vi "Set_Response_Type.vi"(8 "error in (no error)":errorcluster, 11 "OAuth in":refnum<class "OAuth.lvclass">) -> (0 "error out":errorcluster, 3 "OAuth out":refnum<class "OAuth.lvclass">)   [LabVIEW 2016, in "OAuth.lvclass"]
uses:
  OAuth.lvclass
  OAuth.lvclass/OAuth.ctl
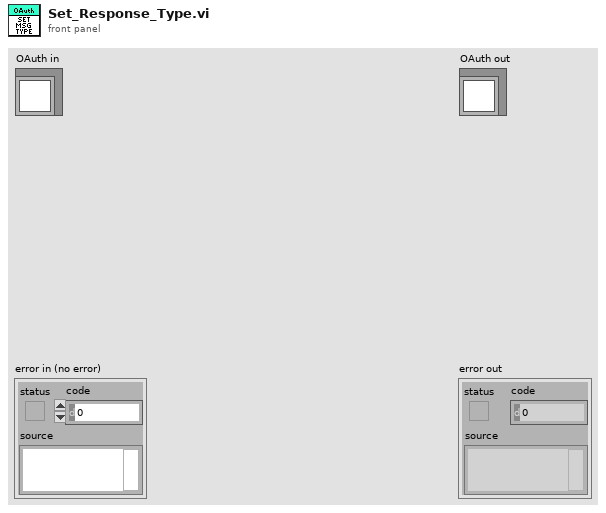
[diagram p1: front panel]
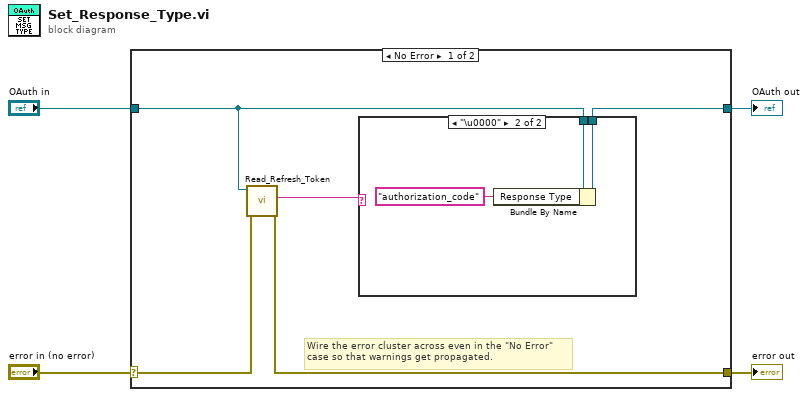
[diagram p0: block diagram]
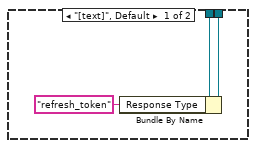
[diagram p2: hidden frame]
diagram:
  n1 = case shown="No Error" "error in (no error)" {
    selector: "error in (no error)" -> [w8 w17]
    tunnel: [w7 w17] -> w3
    tunnel: [w5 w16] -> w1
    tunnel: "OAuth in" -> [w6 w16]
    frame No Error {
      # "Wire the error cluster across even in the \"No Error\"\ncase so that warnings get propagated."
      n2 = call-dynamic "Read_Refresh_Token.vi"("error in (no error)"=w8, "OAuth in"=w6) -> ("error out"=w7:errorcluster, "String"=w9:string)  [unwired: 7 in, 1 out]
      n3 = case shown="\"\"" w9 {
        tunnel: w6 -> [w11 w15]
        tunnel: [w10 w14] -> w5
        frame "[text]", Default {
          n4 = Bundle By Name(cluster=w11, "Response Type"="refresh_token") -> (w10:refnum<class "OAuth.lvclass">)
        }
        frame "\u0000" {
          n5 = Bundle By Name(cluster=w15, "Response Type"="authorization_code") -> (w14:refnum<class "OAuth.lvclass">)
        }
      }
    }
    frame Error {
    }
  }
  "error out" <- w3
  "OAuth out" <- w1
